vi "checkDrop.vi"(8 "error in (no error)":errorcluster, 10 "dragNode in":refnum<data-value>, 11 "dropNode in":refnum<class "xceDataNode.lvclass">) -> (0 "error out":errorcluster, 1 "validDrop":bool, 2 "dragNode out":refnum<data-value>, 3 "dropNode out":refnum<class "xceDataNode.lvclass">)   [LabVIEW 2013, in "xceDataNode.lvclass"]
doc: "Checks to make sure that a drag drop operation is valid. Two conditions must be met:\n1) The drop node must have the drag node's class in its \"allowed subnode[]\" private data.\n2) The drop node must not be a subnode of the drag node."
uses:
  xceDataNode.lvclass
  xceNode/xceNode.lvclass
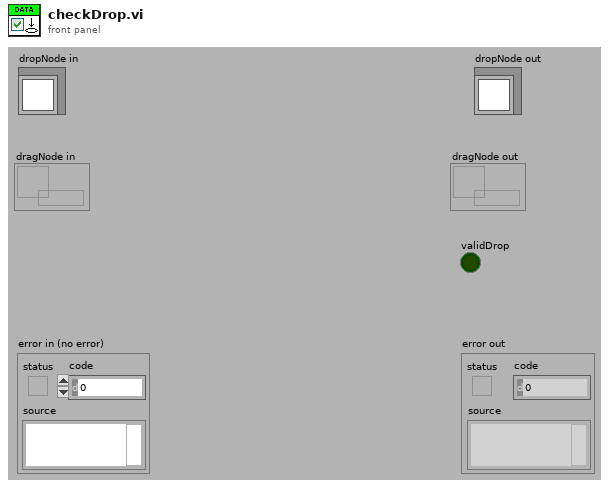
[diagram p1: front panel]
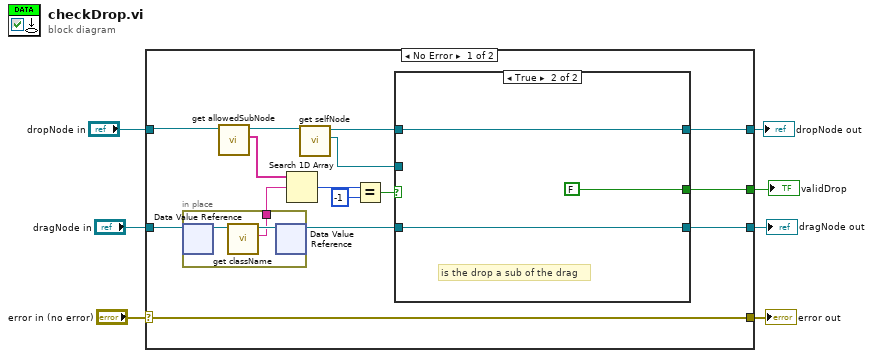
[diagram p0: block diagram]
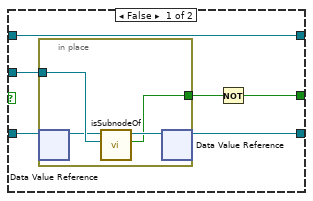
[diagram p2: hidden frame]
diagram:
  n1 = case shown="No Error" "error in (no error)" {
    selector: "error in (no error)" -> [w22 w41]
    tunnel: [w22 w41] -> w6
    tunnel: "dragNode in" -> [w21 w39]
    tunnel: [w16 _] -> w4
    tunnel: "dropNode in" -> [w14 w40]
    tunnel: [w9 w40] -> w2
    tunnel: [w8 w39] -> w1
    frame No Error {
      n2 = in-place {
        in-place-border: [w36] -> w20
        n3 = in-place-dvr #1(w21) -> (w38:refnum<class "xceDataNode.lvclass">)  [unwired: 1 out]
        n4 = call "get className.vi"("xceNode in"=w38) -> ("Class name"=w36:string, "xceNode out"=w37:refnum<class "xceDataNode.lvclass">)  [unwired: 8 in, 1 out]
        n5 = in-place-dvr #1(w37) -> (w10:refnum<data-value>)  [unwired: 1 out]
      }
      n6 = call "get allowedSubNode.vi"("xceDataNode in"=w14) -> ("Allowed subNode[]"=w15:string[], "xceDataNode out"=w13:refnum<class "xceDataNode.lvclass">)  [unwired: 8 in, 1 out]
      n7 = Search 1D Array(1D array=w15, element=w20) -> (index of element=w19:i32)  [unwired: 1 in]
      n8 = call "get selfNode.vi"("xceNode in"=w13) -> ("selfNode*"=w12:refnum<data-value>, "xceNode out"=w11:refnum<class "xceDataNode.lvclass">)  [unwired: 8 in, 1 out]
      n9 = Equal?(x=w19, y=-1) -> (x = y?=w17:bool)
      n10 = case shown="True" w17 {
        tunnel: [w24 FALSE] -> w16
        tunnel: w12 -> [w28 _]
        tunnel: w11 -> [w26 w34]
        tunnel: w10 -> [w27 w33]
        tunnel: [w26 w34] -> w9
        tunnel: [w23 w33] -> w8
        frame False {
          n11 = in-place {
            in-place-border: w28 -> [w32]
            in-place-border: [w29] -> w25
            n12 = in-place-dvr #2(w27) -> (w31:refnum<class "xceDataNode.lvclass">)  [unwired: 1 out]
            n13 = call "isSubnodeOf.vi"("subNode*"=w32, "superNode in"=w31) -> ("isSubNode"=w29:bool, "superNode out"=w30:refnum<class "xceDataNode.lvclass">)  [unwired: 7 in, 1 out]
            n14 = in-place-dvr #2(w30) -> (w23:refnum<data-value>)  [unwired: 1 out]
          }
          n15 = Not(x=w25) -> (.not. x?=w24:bool)
        }
        frame True {
          # "is the drop a sub of the drag"
        }
      }
    }
    frame Error {
    }
  }
  "error out" <- w6
  "validDrop" <- w4
  "dropNode out" <- w2
  "dragNode out" <- w1
